vi "Find Lines.vi"(8 "error in (no error)":errorcluster, 10 "LUT":cluster{u16, u16}, 11 "Image In":T1) -> (0 "error out":errorcluster, 1 "Lines":T2(array[cluster]) {"End Point"."Y" format="%.2f"; "End Point"."X" format="%.2f"; "Start Point"."Y" format="%.2f"; "Start Point"."X" format="%.2f"}, 2 "Number of Matches Returned":i32, 3 "Image Out":T1)   [LabVIEW 2017]
uses:
  <vilib>/vision/Image Controls.llb/IMAQ Image.ctl
  <vilib>/vision/NI_Vision_Development_Module.lvlib
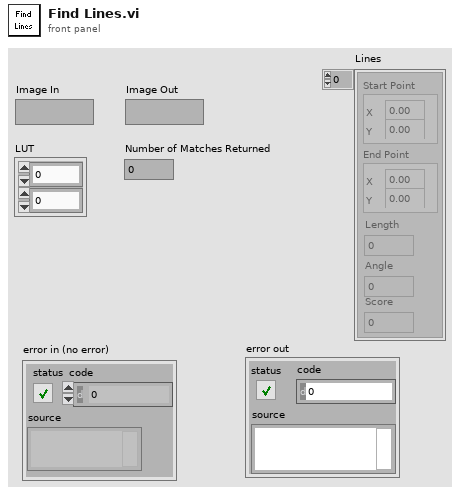
[diagram p1: front panel]
types:
  T1 = typedef "IMAQ Image.ctl" = refnum<image>
  T2 = cluster{"Start Point":cluster{"X":sgl, "Y":sgl}, "End Point":cluster{"X":sgl, "Y":sgl}, "Length":dbl, "Angle":dbl, "Score":dbl}[]
  T3 = typedef "Image Type" = u32
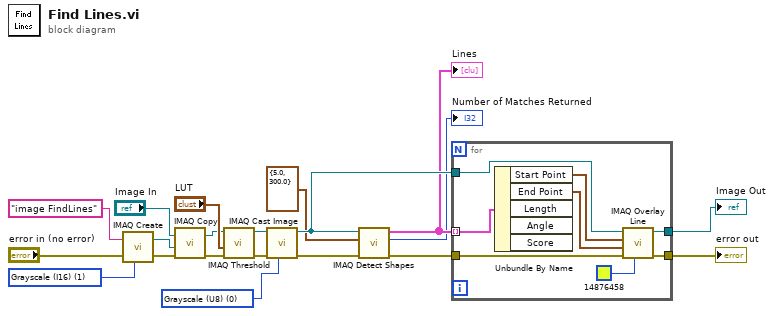
[diagram p0: block diagram]
diagram:
  w15 = T3 0 items=["Grayscale (U8)", "Grayscale (I16)", "Grayscale (SGL)", "Complex (CSG)", "RGB (U32)", "HSL (U32)", "RGB (U64)", "Grayscale (U16)"] ("Image Type")
  w9 = T3 1 items=["Grayscale (U8)", "Grayscale (I16)", "Grayscale (SGL)", "Complex (CSG)", "RGB (U32)", "HSL (U32)", "RGB (U64)", "Grayscale (U16)"] ("Image Type")
  n1 = call "IMAQ Create"("Image Name"="image FindLines", "Image Type"=w9, "error in (no error)"="error in (no error)") -> ("New Image"=w10:T1, "error out"=w1:errorcluster)  [unwired: 2 in]
  n2 = call "IMAQ Copy"("error in (no error)"=w1, "Image Dst"=w10, "Image Src"="Image In") -> ("error out"=w2:errorcluster, "Image Dst Out"=w13:T1)  [unwired: 3 in]
  n3 = call "IMAQ Threshold"("error in (no error)"=w2, "Range"="LUT", "Image Src"=w13) -> ("error out"=w3:errorcluster, "Image Dst Out"=w12:T1)  [unwired: 3 in, 4 out]
  n4 = call "IMAQ Cast Image"("Image Type"=w15, "error in (no error)"=w3, "Image Src"=w12) -> ("error out"=w4:errorcluster, "Image Dst Out"=w19:T1)  [unwired: 7 in]
  n5 = call-poly "IMAQ Detect Shapes"("error in (no error)"=w4, "Line Descriptor"=cluster{"Min Length":dbl, "Max Length":dbl} {"Min Length"=5.0, "Max Length"=300.0}, "Image"=w19) -> ("error out"=w5:errorcluster, "Number of Matches Returned"=→"Number of Matches Returned":i32, "Lines"=w18:T2)  [unwired: 6 in]
  "Lines" <- w18
  n6 = for {
    tunnel: w18 -> [w28] mode=indexing
    tunnel: w19 -> [w27]
    tunnel: [w23] -> w20
    tunnel: [w22] -> w6
    tunnel: w5 -> [w21]
    n7 = Unbundle By Name(w28) -> ("Start Point"=w26:cluster{"X":sgl, "Y":sgl}, "End Point"=w25:cluster{"X":sgl, "Y":sgl})  [unwired: 3 out]
    n8 = call "IMAQ Overlay Line"("Color"=u32 14876458, "error in (no error)"=w21, "End Point"=w25, "Start Point"=w26, "Image"=w27) -> ("error out"=w22:errorcluster, "Image Out"=w23:T1)  [unwired: 5 in]
  }
  "Image Out" <- w20
  "error out" <- w6
